vi "TwGetPeakParametersFromH5.vi"(2 "PeakIndex":i32, 3 "filename":string, 4 "error in (no error)":errorcluster) -> (0 "PeakPar out":T1, 1 "error out":errorcluster)   [LabVIEW 2009]
uses:
  TwH5Dll.dll
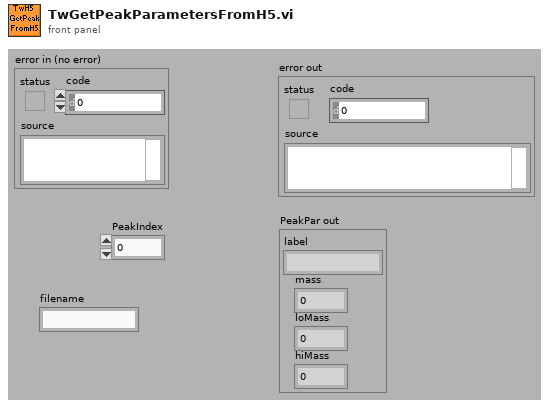
[diagram p1: front panel]
types:
  T1 = cluster{"label":string, "mass":sgl, "loMass":sgl, "hiMass":sgl}
  T2 = cluster{"label":cluster{"[0]":u8, "[1]":u8, "[2]":u8, "[3]":u8, "[4]":u8, "[5]":u8, "[6]":u8, "[7]":u8, "[8]":u8, "[9]":u8, "[10]":u8, "[11]":u8, "[12]":u8, "[13]":u8, "[14]":u8, "[15]":u8, "[16]":u8, "[17]":u8, "[18]":u8, "[19]":u8, "[20]":u8, "[21]":u8, "[22]":u8, "[23]":u8, "[24]":u8, "[25]":u8, "[26]":u8, "[27]":u8, "[28]":u8, "[29]":u8, "[30]":u8, "[31]":u8, "[32]":u8, "[33]":u8, "[34]":u8, "[35]":u8, "[36]":u8, "[37]":u8, "[38]":u8, "[39]":u8, "[40]":u8, "[41]":u8, "[42]":u8, "[43]":u8, "[44]":u8, "[45]":u8, "[46]":u8, "[47]":u8, "[48]":u8, "[49]":u8, "[50]":u8, "[51]":u8, "[52]":u8, "[53]":u8, "[54]":u8, "[55]":u8, "[56]":u8, "[57]":u8, "[58]":u8, "[59]":u8, "[60]":u8, "[61]":u8, "[62]":u8, "[63]":u8}, "mass":sgl, "loMass":sgl, "hiMass":sgl}
  T3 = cluster{"[0]":u8, "[1]":u8, "[2]":u8, "[3]":u8, "[4]":u8, "[5]":u8, "[6]":u8, "[7]":u8, "[8]":u8, "[9]":u8, "[10]":u8, "[11]":u8, "[12]":u8, "[13]":u8, "[14]":u8, "[15]":u8, "[16]":u8, "[17]":u8, "[18]":u8, "[19]":u8, "[20]":u8, "[21]":u8, "[22]":u8, "[23]":u8, "[24]":u8, "[25]":u8, "[26]":u8, "[27]":u8, "[28]":u8, "[29]":u8, "[30]":u8, "[31]":u8, "[32]":u8, "[33]":u8, "[34]":u8, "[35]":u8, "[36]":u8, "[37]":u8, "[38]":u8, "[39]":u8, "[40]":u8, "[41]":u8, "[42]":u8, "[43]":u8, "[44]":u8, "[45]":u8, "[46]":u8, "[47]":u8, "[48]":u8, "[49]":u8, "[50]":u8, "[51]":u8, "[52]":u8, "[53]":u8, "[54]":u8, "[55]":u8, "[56]":u8, "[57]":u8, "[58]":u8, "[59]":u8, "[60]":u8, "[61]":u8, "[62]":u8, "[63]":u8}
  T4 = cluster{"string":string, "mass":sgl, "loMass":sgl, "hiMass":sgl}
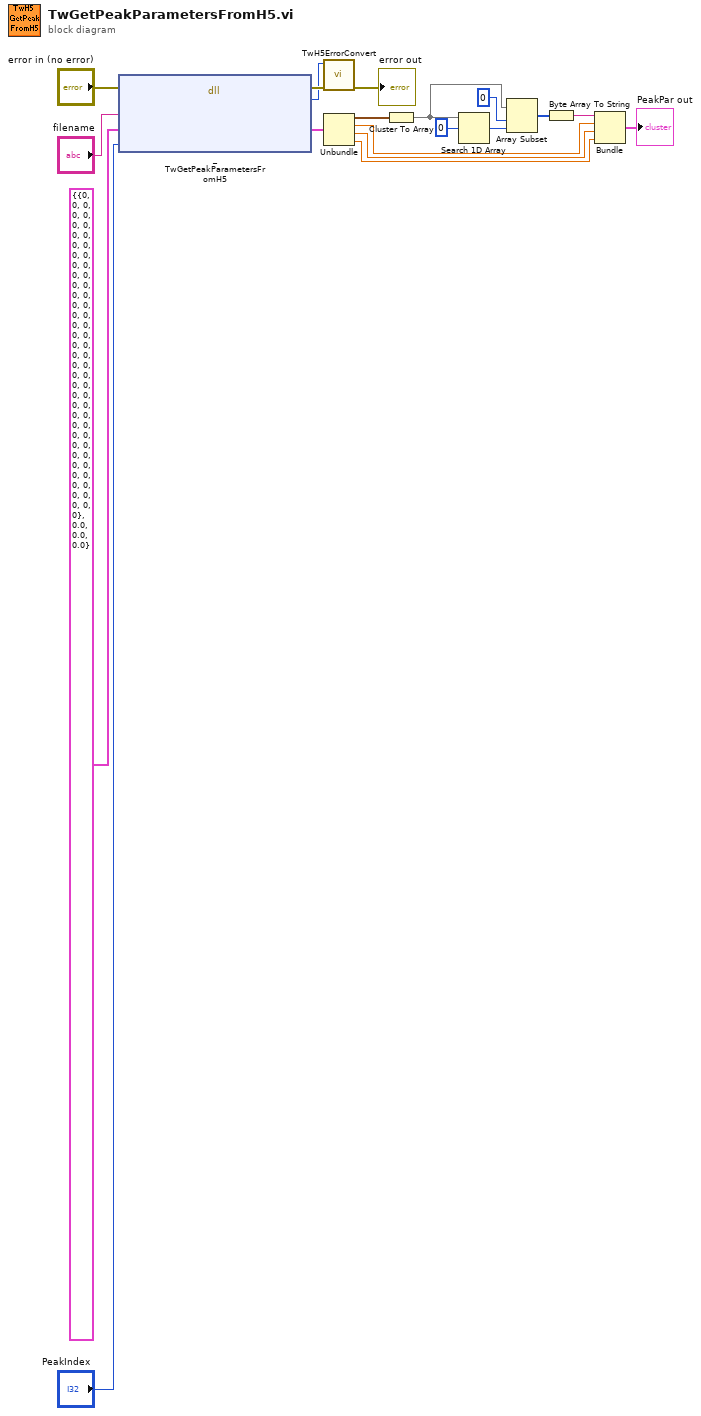
[diagram p0: block diagram]
diagram:
  n1 = dll-call lib="C:/src/85_TofDaq_current/DllWrappers/LabView/TwH5Dll/TwH5Dll.dll" fn="_TwGetPeakParametersFromH5"(error in="error in (no error)", "filename"="filename", "PeakPar"=T2 {"label"={"[0]"=0, "[1]"=0, "[2]"=0, "[3]"=0, "[4]"=0, "[5]"=0, "[6]"=0, "[7]"=0, "[8]"=0, "[9]"=0, "[10]"=0, "[11]"=0, "[12]"=0, "[13]"=0, "[14]"=0, "[15]"=0, "[16]"=0, "[17]"=0, "[18]"=0, "[19]"=0, "[20]"=0, "[21]"=0, "[22]"=0, "[23]"=0, "[24]"=0, "[25]"=0, "[26]"=0, "[27]"=0, "[28]"=0, "[29]"=0, "[30]"=0, "[31]"=0, "[32]"=0, "[33]"=0, "[34]"=0, "[35]"=0, "[36]"=0, "[37]"=0, "[38]"=0, "[39]"=0, "[40]"=0, "[41]"=0, "[42]"=0, "[43]"=0, "[44]"=0, "[45]"=0, "[46]"=0, "[47]"=0, "[48]"=0, "[49]"=0, "[50]"=0, "[51]"=0, "[52]"=0, "[53]"=0, "[54]"=0, "[55]"=0, "[56]"=0, "[57]"=0, "[58]"=0, "[59]"=0, "[60]"=0, "[61]"=0, "[62]"=0, "[63]"=0}, "mass"=0.0, "loMass"=0.0, "hiMass"=0.0} ("peakPar in"), "PeakIndex"="PeakIndex") -> (error out=w18:errorcluster, "TwRetVal"=w17:i32, "PeakPar"=w2:T2)  [unwired: 3 in, 2 out]
  n2 = call "TwH5ErrorConvert.vi"("error in (no error)"=w18, "error code"=w17) -> ("error out"=→"error out":errorcluster)  [unwired: 9 out]
  n3 = Unbundle(w2) -> ("label"=w14:T3, "mass"=w10:sgl, "loMass"=w11:sgl, "hiMass"=w12:sgl)
  n4 = Cluster To Array(cluster=w14) -> (array=w4:u8[])
  n5 = Search 1D Array(1D array=w4, element=u8 0) -> (index of element=w7:i32)  [unwired: 1 out]
  n6 = Array Subset(array=w4, index=0, length=w7) -> (w6:u8[])
  n7 = Byte Array To String(unsigned byte array=w6) -> (string=w3:string)
  n8 = Bundle("string"=w3, "mass"=w10, "loMass"=w11, "hiMass"=w12) -> (→"PeakPar out":T4)  [unwired: 1 out]
